vi "CRYPlot Data.vi"(6 "Down/Right Click?":bool=TRUE, 8 "Visible?":bool=TRUE, 9 "Rows":i32[](array[numeric]), 10 "Graph Type":string="XY", 11 "CurLib Tab Type":enum16{"Curves", "Values", "Results", "WFM"}(ring)) -> ()   [LabVIEW 2013]
uses:
  CRYWindow/DataView/SubVI/CRYData View Global.vi
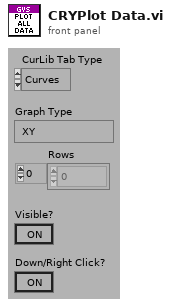
[diagram p1: front panel]
types:
  T1 = enum16{"OK", "Yes", "YesNo", "YesNoCancel", "ReplaceAppend"}
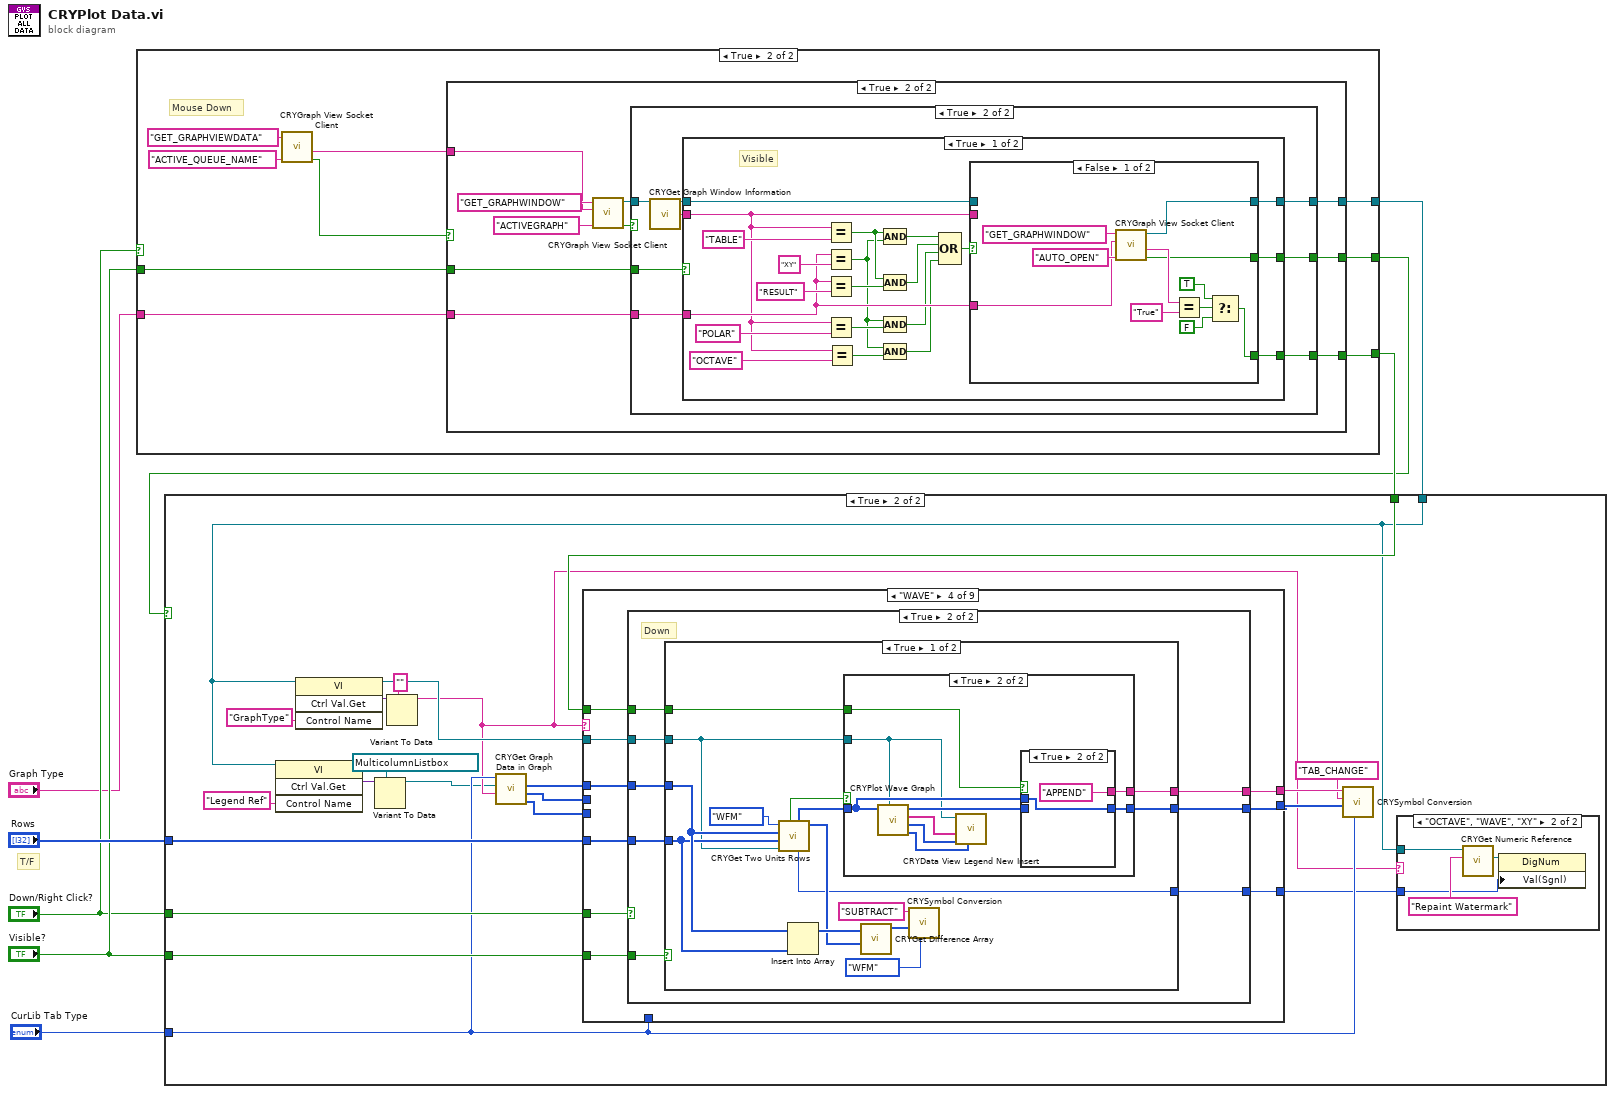
[diagram p0: block diagram]
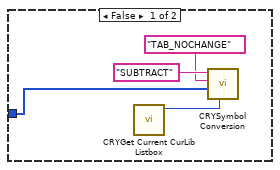
[diagram p2: hidden frame]
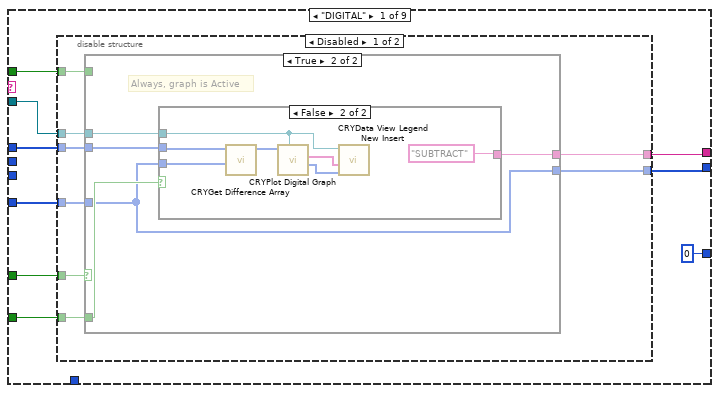
[diagram p4: hidden frame]
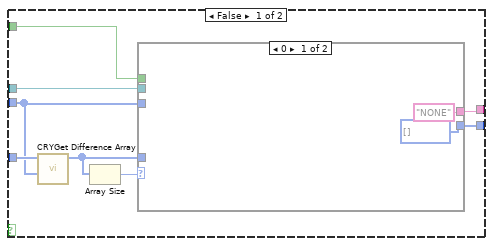
[diagram p5: hidden frame]
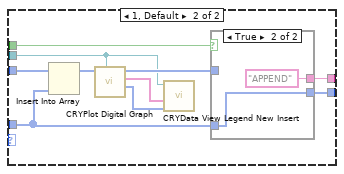
[diagram p6: hidden frame]
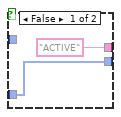
[diagram p7: hidden frame]
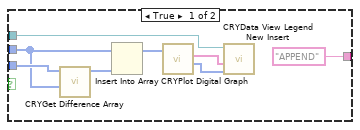
[diagram p8: hidden frame]
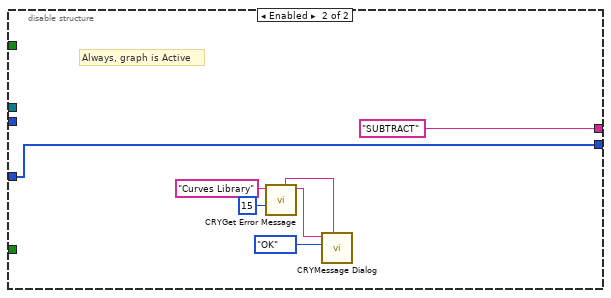
[diagram p9: hidden frame]
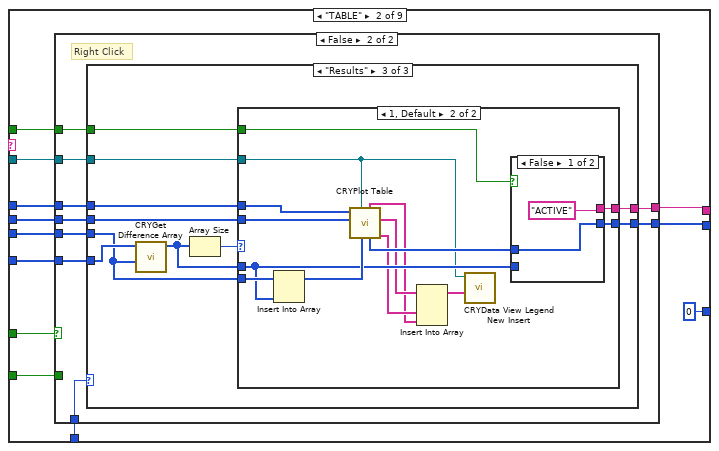
[diagram p10: hidden frame]
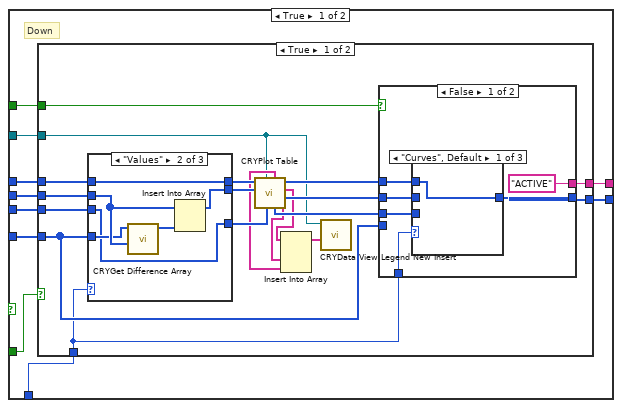
[diagram p11: hidden frame]
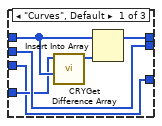
[diagram p12: hidden frame]
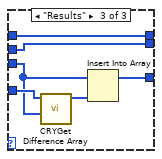
[diagram p13: hidden frame]
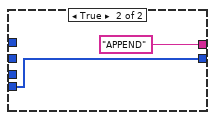
[diagram p16: hidden frame]
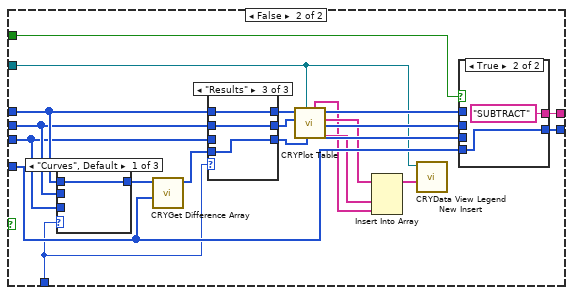
[diagram p17: hidden frame]
diagram:
  # "T/F"
  n1 = case shown="True" "Down/Right Click?" {
    tunnel: "Graph Type" -> [w9 w26]
    tunnel: [w11 w28] -> w5
    tunnel: "Visible?" -> [_ w29]
    tunnel: [w12 w27] -> w6
    tunnel: [w10 w22] -> w2
    frame False {
      # "Right Click"
      n2 = global write "CRYData View Global.vi" "Plot in Right Click?"(TRUE ("Plot in Right Click?")) -> ()
      n3 = call "CRYGraph View Socket Client.vi"("sOption"="AUTO_OPEN", "sData"=w9, "sAction"="GET_GRAPHWINDOW") -> ("bResult Out"=w10:bool, "sData Out"=w13:string, "pVI Out"=w11:refnum<vi>)  [unwired: 5 in, 1 out]
      n4 = Equal?(x=w13, y="True" ("sData Out")) -> (x = y?=w15:bool)
      n5 = Select(t=TRUE, s=w15, f=FALSE) -> (s? t:f=w12:bool)
    }
    frame True {
      # "Mouse Down"
      n6 = call "CRYGraph View Socket Client.vi"("sOption"="ACTIVE_QUEUE_NAME" ("sAction"), "sAction"="GET_GRAPHVIEWDATA") -> ("bResult Out"=w21:bool, "sData Out"=w23:string)  [unwired: 6 in, 2 out]
      n7 = case shown="True" w21 {
        tunnel: w29 -> [_ w50]
        tunnel: [w33 w46] -> w28
        tunnel: [w31 w45] -> w27
        tunnel: w26 -> [w30 w44]
        tunnel: w23 -> [_ w43]
        tunnel: [w32 w41] -> w22
        frame False {
          n8 = call "CRYGraph View Socket Client.vi"("sOption"="AUTO_OPEN", "sData"=w30, "sAction"="GET_GRAPHWINDOW") -> ("bResult Out"=w32:bool, "sData Out"=w34:string, "pVI Out"=w33:refnum<vi>)  [unwired: 5 in, 1 out]
          n9 = Equal?(x=w34, y="True" ("sData Out")) -> (x = y?=w37:bool)
          n10 = Select(t=TRUE, s=w37, f=FALSE) -> (s? t:f=w31:bool)
        }
        frame True {
          n11 = call "CRYGraph View Socket Client.vi"("sOption"="ACTIVEGRAPH", "sData"=w43, "sAction"="GET_GRAPHWINDOW") -> ("bResult Out"=w42:bool, "pVI Out"=w49:refnum<vi>)  [unwired: 5 in, 2 out]
          n12 = case shown="True" w42 {
            tunnel: w50 -> [_ w69]
            tunnel: w49 -> [_ w63]
            tunnel: w44 -> [w51 w67]
            tunnel: [w53 w66] -> w46
            tunnel: [w54 w64] -> w45
            tunnel: [w52 w62] -> w41
            frame False {
              n13 = call "CRYGraph View Socket Client.vi"("sOption"="AUTO_OPEN", "sData"=w51, "sAction"="GET_GRAPHWINDOW") -> ("bResult Out"=w52:bool, "sData Out"=w55:string, "pVI Out"=w53:refnum<vi>)  [unwired: 5 in, 1 out]
              n14 = Equal?(x=w55, y="True" ("sData Out")) -> (x = y?=w58:bool)
              n15 = Select(t=TRUE, s=w58, f=FALSE) -> (s? t:f=w54:bool)
            }
            frame True {
              n16 = call "CRYGet Graph Window Information.vi"("pGraph VI In"=w63) -> ("pGraph VI Out"=w68:refnum<vi>, "Graph Type Out"=w65:string)  [unwired: 2 in, 11 out]
              n17 = case shown="True" w69 {
                tunnel: w67 -> [w77 _]
                tunnel: w65 -> [w74 w107]
                tunnel: [w82 w112] -> w66
                tunnel: w68 -> [w83 w112]
                tunnel: [w81 TRUE] -> w64
                tunnel: [w80 TRUE ("bResult Out")] -> w62
                frame True {
                  # "Visible"
                  n18 = Equal?(x=w74, y="TABLE") -> (x = y?=w86:bool)
                  n19 = Equal?(x=w77, y="XY") -> (x = y?=w73:bool)
                  n20 = Equal?(x=w77, y="RESULT") -> (x = y?=w84:bool)
                  n21 = Equal?(x=w74, y="POLAR") -> (x = y?=w75:bool)
                  n22 = Equal?(x=w74, y="OCTAVE") -> (x = y?=w72:bool)
                  n23 = Compound Arithmetic op=AND(w86, w73) -> (w88:bool)
                  n24 = Compound Arithmetic op=AND(w86, w84) -> (w89:bool)
                  n25 = Compound Arithmetic op=AND(w73, w75) -> (w71:bool)
                  n26 = Compound Arithmetic op=AND(w73, w72) -> (w70:bool)
                  n27 = Compound Arithmetic op=OR(w88, w89, w71, w70) -> (w87:bool)
                  n28 = case shown="False" w87 {
                    tunnel: w77 -> [w91 _]
                    tunnel: [w93 w104] -> w82
                    tunnel: w83 -> [_ w104]
                    tunnel: [w94 w103] -> w81
                    tunnel: [w92 w103] -> w80
                    tunnel: w74 -> [_ w102]
                    frame False {
                      n29 = call "CRYGraph View Socket Client.vi"("sOption"="AUTO_OPEN", "sData"=w91, "sAction"="GET_GRAPHWINDOW") -> ("bResult Out"=w92:bool, "sData Out"=w98:string, "pVI Out"=w93:refnum<vi>)  [unwired: 5 in, 1 out]
                      n30 = Equal?(x=w98, y="True" ("sData Out")) -> (x = y?=w97:bool)
                      n31 = Select(t=TRUE, s=w97, f=FALSE) -> (s? t:f=w94:bool)
                    }
                    frame True {
                      w103 = TRUE
                      n32 = call "CRYGraph View Socket Client.vi"("sOption"="AUTO_OPEN", "sData"=w102, "sAction"="GET_GRAPHWINDOW") -> ()  [unwired: 5 in, 4 out]
                    }
                  }
                }
                frame False {
                  # "Surely, active Window is target to plot"
                  # "Invisible"
                  n33 = call "CRYGraph View Socket Client.vi"("sOption"="AUTO_OPEN", "sData"=w107, "sAction"="GET_GRAPHWINDOW") -> ()  [unwired: 5 in, 4 out]
                }
              }
            }
          }
        }
      }
    }
  }
  n34 = case shown="True" w2 {
    tunnel: "Rows" -> [w114 w138]
    tunnel: "Visible?" -> [_ w137]
    tunnel: w6 -> [_ w136]
    tunnel: w5 -> [_ w118]
    tunnel: "CurLib Tab Type" -> [_ w134]
    tunnel: "Down/Right Click?" -> [_ w135]
    frame False {
      n35 = call "CRYGet Current CurLib Listbox.vi"() -> ("Type"=w113:enum16{"Curves", "Values", "Results", "WFM"})  [unwired: 9 in, 2 out]
      n36 = call "CRYSymbol Conversion.vi"("CurLib Tab Type"=w113, "nDatas"=w114, "sData"="TAB_NOCHANGE" ("sActin"), "sActin"="SUBTRACT") -> ()  [unwired: 8 in]
    }
    frame True {
      n37 = invoke class="VI" method="Ctrl Val.Get"(reference=w118, "Control Name"="Legend Ref") -> ("Get Control Value Variant"=w120:variant)  [unwired: 2 in, 3 out]
      n38 = invoke class="VI" method="Ctrl Val.Get"(reference=w118, "Control Name"="GraphType") -> (reference out=w123:refnum<vi>, "Get Control Value Variant"=w124:variant)  [unwired: 2 in, 2 out]
      n39 = Variant To Data(type=refnum<vi> refnum ("GMListbox"), Variant=w120) -> (data=w117:refnum<vi>)  [unwired: 1 in, 1 out]
      n40 = Variant To Data(type="", Variant=w124) -> (data=w122:string)  [unwired: 1 in, 1 out]
      n41 = call "CRYGet Graph Data in Graph.vi"("Graph Type"=w122, "Legend Refnum"=w117, "Type In"=w134) -> ("Result Rows"=w131:i32[], "Value Rows"=w132:i32[], "Rows"=w133:i32[])  [unwired: 1 in, 5 out]
      n42 = case shown="\"WAVE\"" w122 {
        tunnel: w138 -> [w151 w222 w423 w487 w571 w636 w731 w830 _]
        tunnel: w133 -> [w150 w218 w424 w488 w572 w635 w730 w829 _]
        tunnel: w134 -> [_ w214 _ _ _ _ _ _ _]
        tunnel: w137 -> [w148 w219 w425 w489 w573 w632 w727 w826 _]
        tunnel: w135 -> [w149 w221 w422 w486 w570 w633 w728 w827 _]
        tunnel: w136 -> [w147 w220 w421 w485 _ w634 w729 w828 _]
        tunnel: [0 ("Two Units") 0 ("Two Units") 0 ("Two Units") w481 _ w631 w726 w825 0 ("Two Units")] -> w130
        tunnel: w132 -> [_ w217 _ _ _ _ _ _ _]
        tunnel: w131 -> [_ w215 _ _ _ _ _ _ _]
        tunnel: [w145 w213 w419 w484 w569 w630 w725 w824 "NONE" ("sActin")] -> w129
        tunnel: [w144 w212 w418 w483 w568 w629 w724 w823 i32[] [] ("Rows")] -> w128
        tunnel: w123 -> [w143 w211 w417 w482 w567 w628 w723 w822 _]
        frame "DIGITAL" {
          n43 = disable-structure shown="Disabled" {
            disable-tunnel: w151 -> [w159 w209]
            disable-tunnel: w150 -> [w158 _]
            disable-tunnel: w149 -> [w157 _]
            disable-tunnel: w148 -> [w156 _]
            disable-tunnel: w147 -> [w155 _]
            disable-tunnel: [w154 "SUBTRACT" ("sActin")] -> w145
            disable-tunnel: [w153 w209] -> w144
            disable-tunnel: w143 -> [w152 _]
            frame Disabled {
              n44 = case shown="True" w157 {
                tunnel: w159 -> [w165 w185]
                tunnel: w158 -> [w164 w188]
                tunnel: w156 -> [_ w187]
                tunnel: w155 -> [w163 _]
                tunnel: [w162 w186] -> w154
                tunnel: [w161 w185] -> w153
                tunnel: w152 -> [w160 w184]
                frame False {
                  n45 = call "CRYGet Difference Array.vi"("Array 2"=w164, "Array 1"=w165) -> ("Diff Out"=w167:i32[])  [unwired: 3 in, 6 out]
                  n46 = Array Size(array=w167) -> (size(s)=w166:i32)
                  n47 = case shown="0" w166 {
                    tunnel: w167 -> [_ w177]
                    tunnel: w164 -> [_ w179]
                    tunnel: w163 -> [_ w178]
                    tunnel: ["NONE" ("sActin") w172] -> w162
                    tunnel: [i32[] [] ("Rows") w171] -> w161
                    tunnel: w160 -> [_ w170]
                    frame 0 {
                    }
                    frame 1, Default {
                      n48 = Insert Into Array(array=w179, new element=w177) -> (w174:i32[])  [unwired: 1 in]
                      n49 = call "CRYPlot Digital Graph.vi"("pGraph VI In"=w170, "Selected Row In"=w174) -> ("Color Info"=w175:u32[], "Curve Name"=w176:string[], "Selected Row Out"=w173:i32[])  [unwired: 7 in]
                      n50 = call "CRYData View Legend New Insert.vi"("Color Array"=w175, "ItemName Array"=w176, "pGraph VI In"=w170) -> ()  [unwired: 2 in, 7 out]
                      n51 = case shown="True" w178 {
                        tunnel: w173 -> [_ _]
                        tunnel: w177 -> [w180 w182]
                        tunnel: ["ACTIVE" ("sActin") "APPEND" ("sActin")] -> w172
                        tunnel: [w180 w182] -> w171
                        frame False {
                        }
                        frame True {
                        }
                      }
                    }
                  }
                }
                frame True {
                  # "Always, graph is Active"
                  n52 = case shown="False" w187 {
                    tunnel: w185 -> [w195 w202]
                    tunnel: w188 -> [w194 w203]
                    tunnel: ["APPEND" ("sActin") "SUBTRACT" ("sActin")] -> w186
                    tunnel: w184 -> [w189 w197]
                    frame True {
                      n53 = call "CRYGet Difference Array.vi"("Array 2"=w194, "Array 1"=w195) -> ("Diff Out"=w196:i32[])  [unwired: 3 in, 6 out]
                      n54 = Insert Into Array(array=w194, new element=w196) -> (w191:i32[])  [unwired: 1 in]
                      n55 = call "CRYPlot Digital Graph.vi"("Selected Row In"=w191) -> ("Color Info"=w193:u32[], "Curve Name"=w192:string[])  [unwired: 8 in, 1 out]
                      n56 = call "CRYData View Legend New Insert.vi"("Color Array"=w193, "ItemName Array"=w192, "pGraph VI In"=w189) -> ()  [unwired: 2 in, 7 out]
                    }
                    frame False {
                      n57 = call "CRYGet Difference Array.vi"("Array 2"=w202, "Array 1"=w203) -> ("Diff Out"=w200:i32[])  [unwired: 3 in, 6 out]
                      n58 = call "CRYPlot Digital Graph.vi"("pGraph VI In"=w197, "Selected Row In"=w200) -> ("Color Info"=w199:u32[], "Curve Name"=w201:string[])  [unwired: 7 in, 1 out]
                      n59 = call "CRYData View Legend New Insert.vi"("Color Array"=w199, "ItemName Array"=w201, "pGraph VI In"=w197) -> ()  [unwired: 2 in, 7 out]
                    }
                  }
                }
              }
            }
            frame Enabled {
              # "Always, graph is Active"
              n60 = call "CRYGet Error Message.vi"("Error No"=15, "Kind"="Curves Library") -> ("Message"=w207:string, "Window Title"=w208:string)  [unwired: 4 in, 4 out]
              n61 = call "CRYMessage Dialog.vi"("Window Title"=w208, "YesNoCancel"=T1."OK", "Message Content"=w207) -> ()  [unwired: 7 in, 2 out]
            }
          }
        }
        frame "TABLE" {
          n62 = case shown="False" w221 {
            tunnel: w219 -> [w226 _]
            tunnel: w218 -> [w232 w325]
            tunnel: w222 -> [w230 w326]
            tunnel: w214 -> [w228 w323]
            tunnel: w220 -> [w231 w324]
            tunnel: w217 -> [w229 w322]
            tunnel: w215 -> [w227 w321]
            tunnel: [w225 w320] -> w213
            tunnel: [w224 w319] -> w212
            tunnel: w211 -> [w223 w318]
            frame True {
              # "Down"
              n63 = case shown="True" w226 {
                tunnel: w232 -> [w251 w301]
                tunnel: w231 -> [w250 w300]
                tunnel: w230 -> [w241 w298]
                tunnel: w229 -> [w248 w297]
                tunnel: w228 -> [w240 w286]
                tunnel: w227 -> [w246 w295]
                tunnel: [w239 w287] -> w224
                tunnel: [w238 w288] -> w225
                tunnel: w223 -> [w233 w281]
                frame True {
                  n64 = case shown="\"Values\"" w240 {
                    tunnel: w241 -> [w254 w260 w268]
                    tunnel: [w256 w263 w265] -> w243
                    tunnel: w248 -> [w256 w261 w265]
                    tunnel: [w257 w262 w269] -> w244
                    tunnel: w251 -> [w255 w262 w269]
                    tunnel: w246 -> [w252 w258 w266]
                    tunnel: [w252 w258 w264] -> w242
                    frame "Curves", Default {
                      n65 = call "CRYGet Difference Array.vi"("Array 2"=w255, "Array 1"=w254) -> ("Diff Out"=w253:i32[])  [unwired: 3 in, 6 out]
                      n66 = Insert Into Array(array=w255, new element=w253) -> (w257:i32[])  [unwired: 1 in]
                    }
                    frame "Values" {
                      n67 = call "CRYGet Difference Array.vi"("Array 2"=w261, "Array 1"=w260) -> ("Diff Out"=w259:i32[])  [unwired: 3 in, 6 out]
                      n68 = Insert Into Array(array=w261, new element=w259) -> (w263:i32[])  [unwired: 1 in]
                    }
                    frame "Results" {
                      n69 = call "CRYGet Difference Array.vi"("Array 2"=w266, "Array 1"=w268) -> ("Diff Out"=w267:i32[])  [unwired: 3 in, 6 out]
                      n70 = Insert Into Array(array=w266, new element=w267) -> (w264:i32[])  [unwired: 1 in]
                    }
                  }
                  n71 = call "CRYPlot Table.vi"("Result Rows In"=w242, "pGraph VI In"=w233, "Value Rows In"=w243, "Curve Rows In"=w244) -> ("Value Name"=w235:string[], "Value Rows Out"=w247:i32[], "Curve Name"=w236:string[], "Curve Rows Out"=w249:i32[], "Result Rows Out"=w245:i32[], "Result Name"=w237:string[])  [unwired: 2 in]
                  n72 = Insert Into Array(array=w236, new element #1=w235, new element #2=w237) -> (w234:string[])  [unwired: 1 in]
                  n73 = call "CRYData View Legend New Insert.vi"("ItemName Array"=w234, "pGraph VI In"=w233) -> ()  [unwired: 3 in, 7 out]
                  n74 = case shown="False" w250 {
                    tunnel: w240 -> [w274 _]
                    tunnel: w241 -> [_ w279]
                    tunnel: w249 -> [w275 _]
                    tunnel: w247 -> [w272 _]
                    tunnel: w245 -> [w273 _]
                    tunnel: [w271 w279] -> w239
                    tunnel: ["ACTIVE" ("sActin") "APPEND" ("sActin")] -> w238
                    frame False {
                      n75 = case shown="\"Curves\", Default" w274 {
                        tunnel: w275 -> [w276 _ _]
                        tunnel: w273 -> [_ _ w278]
                        tunnel: w272 -> [_ w277 _]
                        tunnel: [w276 w277 w278] -> w271
                        frame "Curves", Default {
                        }
                        frame "Values" {
                        }
                        frame "Results" {
                        }
                      }
                    }
                    frame True {
                    }
                  }
                }
                frame False {
                  n76 = case shown="\"Curves\", Default" w286 {
                    tunnel: w301 -> [w311 _ _]
                    tunnel: w297 -> [_ w312 _]
                    tunnel: w295 -> [_ _ w313]
                    tunnel: [w311 w312 w313] -> w293
                    frame "Curves", Default {
                    }
                    frame "Values" {
                    }
                    frame "Results" {
                    }
                  }
                  n77 = call "CRYGet Difference Array.vi"("Array 2"=w298, "Array 1"=w293) -> ("Diff Out"=w292:i32[])  [unwired: 3 in, 6 out]
                  n78 = case shown="\"Results\"" w286 {
                    tunnel: w301 -> [_ w306 w309]
                    tunnel: w297 -> [w303 _ w308]
                    tunnel: w295 -> [w302 w305 _]
                    tunnel: [w304 w306 w309] -> w291
                    tunnel: w292 -> [w304 w307 w310]
                    tunnel: [w303 w307 w308] -> w290
                    tunnel: [w302 w305 w310] -> w289
                    frame "Curves", Default {
                    }
                    frame "Values" {
                    }
                    frame "Results" {
                    }
                  }
                  n79 = call "CRYPlot Table.vi"("Result Rows In"=w289, "pGraph VI In"=w281, "Value Rows In"=w290, "Curve Rows In"=w291) -> ("Value Name"=w284:string[], "Value Rows Out"=w296:i32[], "Curve Name"=w285:string[], "Curve Rows Out"=w299:i32[], "Result Rows Out"=w294:i32[], "Result Name"=w283:string[])  [unwired: 2 in]
                  n80 = Insert Into Array(array=w285, new element #1=w284, new element #2=w283) -> (w282:string[])  [unwired: 1 in]
                  n81 = call "CRYData View Legend New Insert.vi"("ItemName Array"=w282, "pGraph VI In"=w281) -> ()  [unwired: 3 in, 7 out]
                  n82 = case shown="True" w300 {
                    tunnel: w298 -> [_ w316]
                    tunnel: w299 -> [_ _]
                    tunnel: w296 -> [_ _]
                    tunnel: w294 -> [_ _]
                    tunnel: ["NONE" ("sActin") "SUBTRACT" ("sActin")] -> w288
                    tunnel: [i32[] [] ("Rows") w316] -> w287
                    frame False {
                    }
                    frame True {
                    }
                  }
                }
              }
            }
            frame False {
              # "Right Click"
              n83 = case shown="\"Results\"" w323 {
                tunnel: w326 -> [w334 w364 w391]
                tunnel: w325 -> [w333 w361 w394]
                tunnel: w324 -> [w332 w363 w395]
                tunnel: w322 -> [w331 w362 w393]
                tunnel: w321 -> [w330 w360 w390]
                tunnel: [w329 w359 w389] -> w320
                tunnel: [w328 w358 w388] -> w319
                tunnel: w318 -> [w327 w357 w387]
                frame "Curves", Default {
                  n84 = call "CRYGet Difference Array.vi"("Array 2"=w333, "Array 1"=w334) -> ("Diff Out"=w335:i32[])  [unwired: 3 in, 6 out]
                  n85 = Array Size(array=w335) -> (size(s)=w336:i32)
                  n86 = case shown="1, Default" w336 {
                    tunnel: w333 -> [_ w349]
                    tunnel: w335 -> [_ w350]
                    tunnel: w332 -> [_ w351]
                    tunnel: w331 -> [_ w347]
                    tunnel: w330 -> [_ w346]
                    tunnel: ["NONE" ("sActin") w345] -> w329
                    tunnel: [i32[] [] ("Rows") w344] -> w328
                    tunnel: w327 -> [_ w339]
                    frame 0 {
                    }
                    frame 1, Default {
                      n87 = Insert Into Array(array=w349, new element=w350) -> (w348:i32[])  [unwired: 1 in]
                      n88 = call "CRYPlot Table.vi"("Result Rows In"=w346, "pGraph VI In"=w339, "Value Rows In"=w347, "Curve Rows In"=w348) -> ("Value Name"=w341:string[], "Curve Name"=w342:string[], "Curve Rows Out"=w352:i32[], "Result Name"=w340:string[])  [unwired: 2 in, 2 out]
                      n89 = Insert Into Array(array=w342, new element #1=w341, new element #2=w340) -> (w343:string[])  [unwired: 1 in]
                      n90 = call "CRYData View Legend New Insert.vi"("ItemName Array"=w343, "pGraph VI In"=w339) -> ()  [unwired: 3 in, 7 out]
                      n91 = case shown="False" w351 {
                        tunnel: w352 -> [w353 _]
                        tunnel: w350 -> [_ w355]
                        tunnel: ["ACTIVE" ("sActin") "APPEND" ("sActin")] -> w345
                        tunnel: [w353 w355] -> w344
                        frame False {
                        }
                        frame True {
                        }
                      }
                    }
                  }
                }
                frame "Values" {
                  n92 = call "CRYGet Difference Array.vi"("Array 2"=w362, "Array 1"=w364) -> ("Diff Out"=w365:i32[])  [unwired: 3 in, 6 out]
                  n93 = Array Size(array=w365) -> (size(s)=w366:i32)
                  n94 = case shown="1, Default" w366 {
                    tunnel: w362 -> [_ w380]
                    tunnel: w365 -> [_ w381]
                    tunnel: w363 -> [_ w382]
                    tunnel: w361 -> [_ w378]
                    tunnel: w360 -> [_ w376]
                    tunnel: ["NONE" ("sActin") w375] -> w359
                    tunnel: [i32[] [] ("Rows") w374] -> w358
                    tunnel: w357 -> [_ w369]
                    frame 0 {
                    }
                    frame 1, Default {
                      n95 = Insert Into Array(array=w380, new element=w381) -> (w379:i32[])  [unwired: 1 in]
                      n96 = call "CRYPlot Table.vi"("Result Rows In"=w376, "pGraph VI In"=w369, "Value Rows In"=w379, "Curve Rows In"=w378) -> ("Value Name"=w371:string[], "Value Rows Out"=w377:i32[], "Curve Name"=w372:string[], "Result Name"=w370:string[])  [unwired: 2 in, 2 out]
                      n97 = Insert Into Array(array=w372, new element #1=w371, new element #2=w370) -> (w373:string[])  [unwired: 1 in]
                      n98 = call "CRYData View Legend New Insert.vi"("ItemName Array"=w373, "pGraph VI In"=w369) -> ()  [unwired: 3 in, 7 out]
                      n99 = case shown="False" w382 {
                        tunnel: w381 -> [_ w385]
                        tunnel: w377 -> [w383 _]
                        tunnel: ["ACTIVE" ("sActin") "APPEND" ("sActin")] -> w375
                        tunnel: [w383 w385] -> w374
                        frame False {
                        }
                        frame True {
                        }
                      }
                    }
                  }
                }
                frame "Results" {
                  n100 = call "CRYGet Difference Array.vi"("Array 2"=w390, "Array 1"=w391) -> ("Diff Out"=w392:i32[])  [unwired: 3 in, 6 out]
                  n101 = Array Size(array=w392) -> (size(s)=w396:i32)
                  n102 = case shown="1, Default" w396 {
                    tunnel: w392 -> [_ w406]
                    tunnel: w395 -> [_ w412]
                    tunnel: w394 -> [_ w411]
                    tunnel: w393 -> [_ w410]
                    tunnel: w390 -> [_ w409]
                    tunnel: ["NONE" ("sActin") w405] -> w389
                    tunnel: [i32[] [] ("Rows") w404] -> w388
                    tunnel: w387 -> [_ w399]
                    frame 0 {
                    }
                    frame 1, Default {
                      n103 = Insert Into Array(array=w409, new element=w406) -> (w408:i32[])  [unwired: 1 in]
                      n104 = call "CRYPlot Table.vi"("Result Rows In"=w408, "pGraph VI In"=w399, "Value Rows In"=w410, "Curve Rows In"=w411) -> ("Value Name"=w401:string[], "Curve Name"=w402:string[], "Result Rows Out"=w407:i32[], "Result Name"=w400:string[])  [unwired: 2 in, 2 out]
                      n105 = Insert Into Array(array=w402, new element #1=w401, new element #2=w400) -> (w403:string[])  [unwired: 1 in]
                      n106 = call "CRYData View Legend New Insert.vi"("ItemName Array"=w403, "pGraph VI In"=w399) -> ()  [unwired: 3 in, 7 out]
                      n107 = case shown="False" w412 {
                        tunnel: w407 -> [w413 _]
                        tunnel: w406 -> [_ w415]
                        tunnel: ["ACTIVE" ("sActin") "APPEND" ("sActin")] -> w405
                        tunnel: [w413 w415] -> w404
                        frame False {
                        }
                        frame True {
                        }
                      }
                    }
                  }
                }
              }
            }
          }
        }
        frame "RESULT" {
          n108 = case shown="True" w422 {
            tunnel: w425 -> [_ w449]
            tunnel: w424 -> [w431 w454]
            tunnel: w423 -> [w430 w452]
            tunnel: w421 -> [w429 w453]
            tunnel: [w427 w451] -> w418
            tunnel: [w428 w450] -> w419
            tunnel: w417 -> [w426 w448]
            frame False {
              n109 = call "CRYGet Difference Array.vi"("Array 2"=w431, "Array 1"=w430) -> ("Diff Out"=w433:i32[])  [unwired: 3 in, 6 out]
              n110 = Array Size(array=w433) -> (size(s)=w432:i32)
              n111 = case shown="1, Default" w432 {
                tunnel: w431 -> [_ w441]
                tunnel: w433 -> [_ w440]
                tunnel: w429 -> [_ w442]
                tunnel: ["NONE" ("sActin") w439] -> w428
                tunnel: [i32[] [] ("Rows") w438] -> w427
                tunnel: w426 -> [_ w436]
                frame 0 {
                }
                frame 1, Default {
                  n112 = call "CRYPlot Result.vi"("pGraph VI In"=w436, "New Rows In"=w440, "Old Rows In"=w441) -> ("Curve Name"=w437:string[], "Selected Rows Out"=w443:i32[])  [unwired: 2 in, 5 out]
                  n113 = call "CRYData View Legend New Insert.vi"("ItemName Array"=w437, "pGraph VI In"=w436) -> ()  [unwired: 3 in, 7 out]
                  n114 = case shown="False" w442 {
                    tunnel: w443 -> [w444 _]
                    tunnel: w440 -> [_ w446]
                    tunnel: ["ACTIVE" ("sActin") "APPEND" ("sActin")] -> w439
                    tunnel: [w444 w446] -> w438
                    frame False {
                    }
                    frame True {
                    }
                  }
                }
              }
            }
            frame True {
              # "Down"
              n115 = case shown="False" w449 {
                tunnel: w454 -> [w462 w475]
                tunnel: w453 -> [w461 w474]
                tunnel: w452 -> [w460 w473]
                tunnel: [w459 w472] -> w451
                tunnel: [w458 w471] -> w450
                tunnel: w448 -> [w455 w469]
                frame True {
                  n116 = call "CRYGet Difference Array.vi"("Array 2"=w462, "Array 1"=w460) -> ("Diff Out"=w457:i32[])  [unwired: 3 in, 6 out]
                  n117 = Insert Into Array(array=w462, new element=w457) -> (w464:i32[])  [unwired: 1 in]
                  n118 = call "CRYPlot Result.vi"("pGraph VI In"=w455, "Old Rows In"=w464) -> ("Curve Name"=w456:string[], "Selected Rows Out"=w463:i32[])  [unwired: 3 in, 5 out]
                  n119 = call "CRYData View Legend New Insert.vi"("ItemName Array"=w456, "pGraph VI In"=w455) -> ()  [unwired: 3 in, 7 out]
                  n120 = case shown="True" w461 {
                    tunnel: w463 -> [w466 _]
                    tunnel: [w466 w467] -> w459
                    tunnel: ["ACTIVE" ("sActin") "APPEND" ("sActin")] -> w458
                    tunnel: w460 -> [_ w467]
                    frame False {
                    }
                    frame True {
                    }
                  }
                }
                frame False {
                  # "Invisible"
                  n121 = call "CRYGet Difference Array.vi"("Array 2"=w473, "Array 1"=w475) -> ("Diff Out"=w476:i32[])  [unwired: 3 in, 6 out]
                  n122 = call "CRYPlot Result.vi"("pGraph VI In"=w469, "Old Rows In"=w476) -> ("Curve Name"=w470:string[])  [unwired: 3 in, 6 out]
                  n123 = call "CRYData View Legend New Insert.vi"("ItemName Array"=w470, "pGraph VI In"=w469) -> ()  [unwired: 3 in, 7 out]
                  n124 = case shown="True" w474 {
                    tunnel: [i32[] [] ("Rows") w479] -> w472
                    tunnel: ["NONE" ("sActin") "SUBTRACT" ("sActin")] -> w471
                    tunnel: w473 -> [_ w479]
                    frame False {
                    }
                    frame True {
                    }
                  }
                }
              }
            }
          }
        }
        frame "WAVE" {
          n125 = case shown="True" w486 {
            tunnel: w489 -> [_ w517]
            tunnel: w488 -> [w493 w522]
            tunnel: w487 -> [w492 w520]
            tunnel: w485 -> [w499 w521]
            tunnel: [w498 w519] -> w483
            tunnel: [w497 w518] -> w484
            tunnel: w482 -> [w490 w516]
            tunnel: [w491 w515] -> w481
            frame False {
              n126 = call "CRYGet Two Units Rows.vi"("pGraph VI In"=w490, "New Rows In"=w492, "Old Rows In"=w493, "Type"=enum16{"Curves", "Values", "Results", "WFM"}."WFM") -> ("Two Units"=w491:i32, "New Rows Out"=w495:i32[], "New Exist?"=w496:bool)  [unwired: 1 in, 4 out]
              n127 = case shown="True" w496 {
                tunnel: w493 -> [_ _]
                tunnel: w495 -> [w502 _]
                tunnel: w499 -> [w505 _]
                tunnel: [w503 i32[] [] ("Rows")] -> w498
                tunnel: [w504 "NONE" ("sActin")] -> w497
                tunnel: w490 -> [w500 _]
                frame True {
                  n128 = call "CRYPlot Wave Graph.vi"("pGraph VI In"=w500, "Selected Rows In"=w502) -> ("ItemSyms"=w501:i32[], "Color Info"=w508:u32[], "Curve Name"=w507:string[], "Selected Rows Out"=w506:i32[])  [unwired: 3 in, 3 out]
                  n129 = call "CRYData View Legend New Insert.vi"("Item Symbols"=w501, "Color Array"=w508, "ItemName Array"=w507, "pGraph VI In"=w500) -> ()  [unwired: 1 in, 7 out]
                  n130 = case shown="False" w505 {
                    tunnel: w506 -> [w509 _]
                    tunnel: w502 -> [_ w511]
                    tunnel: ["ACTIVE" ("sActin") "APPEND" ("sActin")] -> w504
                    tunnel: [w509 w511] -> w503
                    frame False {
                    }
                    frame True {
                    }
                  }
                }
                frame False {
                }
              }
            }
            frame True {
              # "Down"
              n131 = case shown="True" w517 {
                tunnel: w522 -> [w528 w556]
                tunnel: w521 -> [w537 _]
                tunnel: w520 -> [w527 w555]
                tunnel: [w536 i32[] [] ("Rows")] -> w519
                tunnel: [w535 "NONE" ("sActin")] -> w518
                tunnel: w516 -> [w524 w559]
                tunnel: [w525 0 ("Two Units")] -> w515
                frame True {
                  n132 = call "CRYGet Two Units Rows.vi"("pGraph VI In"=w524, "New Rows In"=w527, "Old Rows In"=w528, "Type"=enum16{"Curves", "Values", "Results", "WFM"}."WFM") -> ("All Rows Out"=w526:i32[], "Two Units"=w525:i32, "New Rows Out"=w533:i32[], "New Exist?"=w534:bool)  [unwired: 1 in, 3 out]
                  n133 = Insert Into Array(array=w528, new element=w527) -> (w529:i32[])  [unwired: 1 in]
                  n134 = case shown="True" w534 {
                    tunnel: w537 -> [_ w545]
                    tunnel: [i32[] [] ("New Rows Out") w544] -> w536
                    tunnel: ["NONE" ("sActin") w543] -> w535
                    tunnel: w533 -> [_ w541]
                    tunnel: w524 -> [_ w540]
                    frame False {
                    }
                    frame True {
                      n135 = call "CRYPlot Wave Graph.vi"("pGraph VI In"=w540, "Selected Rows In"=w541) -> ("ItemSyms"=w542:i32[], "Color Info"=w546:u32[], "Curve Name"=w547:string[], "Selected Rows Out"=w548:i32[])  [unwired: 3 in, 3 out]
                      n136 = call "CRYData View Legend New Insert.vi"("Item Symbols"=w542, "Color Array"=w546, "ItemName Array"=w547, "pGraph VI In"=w540) -> ()  [unwired: 1 in, 7 out]
                      n137 = case shown="True" w545 {
                        tunnel: w548 -> [w550 _]
                        tunnel: [w550 w551] -> w544
                        tunnel: ["ACTIVE" ("sActin") "APPEND" ("sActin")] -> w543
                        tunnel: w541 -> [_ w551]
                        frame False {
                        }
                        frame True {
                        }
                      }
                    }
                  }
                  n138 = call "CRYGet Difference Array.vi"("Array 2"=w526, "Array 1"=w529) -> ("Diff Out"=w530:i32[])  [unwired: 3 in, 6 out]
                  n139 = call "CRYSymbol Conversion.vi"("CurLib Tab Type"=enum16{"Curves", "Values", "Results", "WFM"}."WFM", "nDatas"=w530, "sActin"="SUBTRACT") -> ()  [unwired: 9 in]
                }
                frame False {
                  # "Invisible"
                  n140 = Index Array(array=w555) -> (element=w562:i32)  [unwired: 1 in]
                  n141 = Search 1D Array(1D array=w556, element=w562) -> (index of element=w560:i32)  [unwired: 1 in]
                  n142 = Build Array(w560) -> (w553:i32[])
                  n143 = invoke class="VI" method="Ctrl Val.Set"(reference=w559, "Control Name"="SelectedRow", "Value"=w553) -> (reference out=w566:refnum<vi>)  [unwired: 2 in, 4 out]
                  n144 = call "CRYGet Boolean Reference.vi"("Label Name"="RemoveSome", "VI Refnum"=w566) -> ("Boolean Ref"=w564:refnum<vi>)  [unwired: 7 in, 2 out]
                  n145 = property class="Bool"(reference=w564, "Val(Sgnl)"=TRUE) -> ()  [unwired: 1 in, 2 out]
                }
              }
            }
          }
        }
        frame "INTENSITY" {
          n146 = case shown="True" w570 {
            tunnel: w573 -> [_ w593]
            tunnel: w572 -> [w577 w597]
            tunnel: w571 -> [w578 w596]
            tunnel: [w580 w595] -> w568
            tunnel: [w579 w594] -> w569
            tunnel: w567 -> [w574 w592]
            frame False {
              n147 = call "CRYGet Difference Array.vi"("Array 2"=w577, "Array 1"=w578) -> ("Diff Out"=w575:i32[])  [unwired: 3 in, 6 out]
              n148 = Array Size(array=w575) -> (size(s)=w576:i32)
              n149 = case shown="1, Default" w576 {
                tunnel: [i32[] [] ("All Rows Out") w591] -> w580
                tunnel: ["NONE" ("sActin") "ACTIVE" ("sActin")] -> w579
                tunnel: w577 -> [_ w585]
                tunnel: w575 -> [_ w584]
                tunnel: w574 -> [_ w583]
                frame 0 {
                }
                frame 1, Default {
                  n150 = Insert Into Array(array=w585, new element=w584) -> (w586:i32[])  [unwired: 1 in]
                  n151 = call "CRYPlot Intensity Graph.vi"("pGraph VI In"=w583, "Selected Rows In"=w586) -> ("ItemSyms"=w587:i32[], "Color Info"=w589:u32[], "Wave Names"=w588:string[], "All Rows Out"=w591:i32[])  [unwired: 6 in]
                  n152 = call "CRYData View Legend New Insert.vi"("Item Symbols"=w587, "Color Array"=w589, "ItemName Array"=w588, "pGraph VI In"=w583) -> ()  [unwired: 1 in, 7 out]
                }
              }
            }
            frame True {
              # "Down"
              n153 = case shown="True" w593 {
                tunnel: w597 -> [w601 w618]
                tunnel: w596 -> [w602 w617]
                tunnel: [w604 i32[] [] ("Rows")] -> w595
                tunnel: [w603 "NONE" ("sActin")] -> w594
                tunnel: w592 -> [w598 w621]
                frame True {
                  n154 = call "CRYGet Difference Array.vi"("Array 2"=w601, "Array 1"=w602) -> ("Diff Out"=w599:i32[])  [unwired: 3 in, 6 out]
                  n155 = Array Size(array=w599) -> (size(s)=w600:i32)
                  n156 = case shown="1, Default" w600 {
                    tunnel: [i32[] [] ("All Rows Out") w615] -> w604
                    tunnel: ["NONE" ("sActin") "ACTIVE" ("sActin")] -> w603
                    tunnel: w601 -> [_ w613]
                    tunnel: w599 -> [_ w612]
                    tunnel: w598 -> [_ w607]
                    frame 0 {
                    }
                    frame 1, Default {
                      n157 = Insert Into Array(array=w613, new element=w612) -> (w611:i32[])  [unwired: 1 in]
                      n158 = call "CRYPlot Intensity Graph.vi"("pGraph VI In"=w607, "Selected Rows In"=w611) -> ("ItemSyms"=w608:i32[], "Color Info"=w609:u32[], "Wave Names"=w610:string[], "All Rows Out"=w615:i32[])  [unwired: 6 in]
                      n159 = call "CRYData View Legend New Insert.vi"("Item Symbols"=w608, "Color Array"=w609, "ItemName Array"=w610, "pGraph VI In"=w607) -> ()  [unwired: 1 in, 7 out]
                    }
                  }
                }
                frame False {
                  # "Invisible"
                  n160 = Index Array(array=w617) -> (element=w623:i32)  [unwired: 1 in]
                  n161 = Search 1D Array(1D array=w618, element=w623) -> (index of element=w616:i32)  [unwired: 1 in]
                  n162 = invoke class="VI" method="Ctrl Val.Set"(reference=w621, "Control Name"="OldRow", "Value"=w616) -> (reference out=w627:refnum<vi>)  [unwired: 2 in, 4 out]
                  n163 = call "CRYGet Boolean Reference.vi"("Label Name"="RemoveOne", "VI Refnum"=w627) -> ("Boolean Ref"=w625:refnum<vi>)  [unwired: 7 in, 2 out]
                  n164 = property class="Bool"(reference=w625, "Val(Sgnl)"=TRUE) -> ()  [unwired: 1 in, 2 out]
                }
              }
            }
          }
        }
        frame "XY" {
          n165 = case shown="True" w633 {
            tunnel: w636 -> [w642 w703]
            tunnel: w635 -> [w643 w702]
            tunnel: w634 -> [w641 w707]
            tunnel: w632 -> [w644 _]
            tunnel: [w640 w701] -> w631
            tunnel: [w639 w700] -> w630
            tunnel: [w638 w699] -> w629
            tunnel: w628 -> [w637 w698]
            frame True {
              # "Down"
              n166 = case shown="True" w644 {
                tunnel: w643 -> [w648 w684]
                tunnel: w642 -> [w647 w690]
                tunnel: w641 -> [w657 _]
                tunnel: [w654 w697] -> w640
                tunnel: [w653 "NONE" ("sActin")] -> w639
                tunnel: [w652 i32[] [] ("Rows")] -> w638
                tunnel: w637 -> [w645 w674]
                frame True {
                  n167 = call "CRYGet Two Units Rows.vi"("pGraph VI In"=w645, "New Rows In"=w647, "Old Rows In"=w648) -> ("All Rows Out"=w646:i32[], "Two Units"=w654:i32, "New Rows Out"=w655:i32[], "New Exist?"=w656:bool)  [unwired: 2 in, 3 out]
                  n168 = Insert Into Array(array=w648, new element=w647) -> (w649:i32[])  [unwired: 1 in]
                  n169 = call "CRYGet Difference Array.vi"("Array 2"=w646, "Array 1"=w649) -> ("Diff Out"=w650:i32[])  [unwired: 3 in, 6 out]
                  n170 = case shown="True" w656 {
                    tunnel: w657 -> [w664 _]
                    tunnel: w655 -> [w660 _]
                    tunnel: w647 -> [_ _]
                    tunnel: [w662 "NONE" ("sActin")] -> w653
                    tunnel: [w661 i32[] [] ("New Rows Out")] -> w652
                    tunnel: w645 -> [w658 _]
                    frame True {
                      n171 = call "CRYPlot XY Graph.vi"("pGraph VI In"=w658, "Selected Rows In"=w660) -> ("Color Info"=w666:u32[], "Curve Name"=w665:string[], "All Rows Out"=w663:i32[], "ItemSyms"=w659:i32[])  [unwired: 4 in, 2 out]
                      n172 = call "CRYData View Legend New Insert.vi"("Item Symbols"=w659, "Color Array"=w666, "ItemName Array"=w665, "pGraph VI In"=w658) -> ()  [unwired: 1 in, 7 out]
                      n173 = case shown="False" w664 {
                        tunnel: w663 -> [w668 _]
                        tunnel: w660 -> [_ w669]
                        tunnel: ["ACTIVE" ("sActin") "APPEND" ("sActin")] -> w662
                        tunnel: [w668 w669] -> w661
                        frame False {
                        }
                        frame True {
                        }
                      }
                    }
                    frame False {
                    }
                  }
                  n174 = call "CRYSymbol Conversion.vi"("nDatas"=w650, "sActin"="SUBTRACT") -> ()  [unwired: 10 in]
                }
                frame False {
                  n175 = Index Array(array=w690) -> (element=w689:i32)  [unwired: 1 in]
                  n176 = invoke class="VI" method="Ctrl Val.Get"(reference=w674, "Control Name"="MagnitudeShow") -> ("Get Control Value Variant"=w676:variant)  [unwired: 2 in, 3 out]
                  n177 = invoke class="VI" method="Ctrl Val.Get"(reference=w674, "Control Name"="PhaseShow") -> ("Get Control Value Variant"=w679:variant)  [unwired: 2 in, 3 out]
                  n178 = Variant To Data(type=TRUE, Variant=w676) -> (data=w681:bool)  [unwired: 1 in, 1 out]
                  n179 = Variant To Data(type=TRUE, Variant=w679) -> (data=w682:bool)  [unwired: 1 in, 1 out]
                  n180 = And(x=w681, y=w682) -> (x .and. y?=w673:bool)
                  n181 = call "CRYMake Phase Index.vi"("Mag_Phase Flag"=w673, "Selected Rows In"=w684) -> ("Selected Rows Out"=w683:i32[])  [unwired: 8 in, 1 out]
                  n182 = Search 1D Array(1D array=w683, element=w689) -> (index of element=w687:i32)  [unwired: 1 in]
                  n183 = Build Array(w687) -> (w685:i32[])
                  n184 = invoke class="VI" method="Ctrl Val.Set"(reference=w674, "Control Name"="SelectedRow", "Value"=w685) -> (reference out=w694:refnum<vi>)  [unwired: 2 in, 4 out]
                  n185 = Delete From Array(array=w683, index=w687) -> (array with subset deleted=w686:i32[])  [unwired: 1 in, 1 out]
                  n186 = call "CRYGet Two Units Rows.vi"("pGraph VI In"=w674, "Old Rows In"=w686) -> ("Two Units"=w697:i32)  [unwired: 3 in, 6 out]
                  n187 = call "CRYGet Boolean Reference.vi"("Label Name"="RemoveSome", "VI Refnum"=w694) -> ("Boolean Ref"=w692:refnum<vi>)  [unwired: 7 in, 2 out]
                  n188 = property class="Bool"(reference=w692, "Val(Sgnl)"=TRUE) -> ()  [unwired: 1 in, 2 out]
                }
              }
            }
            frame False {
              n189 = call "CRYGet Difference Array.vi"("Array 2"=w702, "Array 1"=w703) -> ("Diff Out"=w704:i32[])  [unwired: 3 in, 6 out]
              n190 = call "CRYGet Two Units Rows.vi"("pGraph VI In"=w698, "New Rows In"=w704, "Old Rows In"=w702) -> ("Two Units"=w701:i32, "New Rows Out"=w705:i32[], "New Exist?"=w706:bool)  [unwired: 2 in, 4 out]
              n191 = case shown="True" w706 {
                tunnel: w707 -> [_ w718]
                tunnel: w705 -> [_ w712]
                tunnel: ["NONE" ("sActin") w714] -> w700
                tunnel: [i32[] [] ("All Rows Out") w713] -> w699
                tunnel: w698 -> [_ w710]
                frame False {
                }
                frame True {
                  n192 = call "CRYPlot XY Graph.vi"("pGraph VI In"=w710, "Selected Rows In"=w712) -> ("Color Info"=w717:u32[], "Curve Name"=w716:string[], "All Rows Out"=w715:i32[], "ItemSyms"=w711:i32[])  [unwired: 4 in, 2 out]
                  n193 = call "CRYData View Legend New Insert.vi"("Item Symbols"=w711, "Color Array"=w717, "ItemName Array"=w716, "pGraph VI In"=w710) -> ()  [unwired: 1 in, 7 out]
                  n194 = case shown="False" w718 {
                    tunnel: w712 -> [w719 _]
                    tunnel: w715 -> [_ w722]
                    tunnel: ["APPEND" ("sActin") "ACTIVE" ("sActin")] -> w714
                    tunnel: [w719 w722] -> w713
                    frame True {
                    }
                    frame False {
                    }
                  }
                }
              }
            }
          }
        }
        frame "POLAR" {
          n195 = case shown="False" w728 {
            tunnel: w731 -> [w737 w797]
            tunnel: w730 -> [w738 w796]
            tunnel: w729 -> [w736 w801]
            tunnel: w727 -> [w739 _]
            tunnel: [w735 w795] -> w726
            tunnel: [w734 w794] -> w725
            tunnel: [w733 w793] -> w724
            tunnel: w723 -> [w732 w791]
            frame True {
              # "Down"
              n196 = case shown="False" w739 {
                tunnel: w738 -> [w743 w781]
                tunnel: w737 -> [w742 w784]
                tunnel: w736 -> [w752 _]
                tunnel: [w749 w790] -> w735
                tunnel: [w748 "NONE" ("sActin")] -> w734
                tunnel: [w747 i32[] [] ("Rows")] -> w733
                tunnel: w732 -> [w740 w775]
                frame True {
                  n197 = Insert Into Array(array=w743, new element=w742) -> (w744:i32[])  [unwired: 1 in]
                  n198 = call "CRYGet Two Units Rows.vi"("pGraph VI In"=w740, "New Rows In"=w742, "Old Rows In"=w743) -> ("All Rows Out"=w741:i32[], "Two Units"=w749:i32, "New Rows Out"=w750:i32[], "New Exist?"=w751:bool)  [unwired: 2 in, 3 out]
                  n199 = case shown="True" w751 {
                    tunnel: w752 -> [w764 _]
                    tunnel: w750 -> [w756 _]
                    tunnel: w742 -> [_ _]
                    tunnel: [w762 "NONE" ("sActin")] -> w748
                    tunnel: [w761 i32[] [] ("New Rows Out")] -> w747
                    tunnel: w741 -> [w755 _]
                    tunnel: w740 -> [w754 _]
                    frame True {
                      w753 = "POLAR_PlotXY" ("sOption")
                      n200 = call "CRYPlot XY Graph.vi"("pGraph VI In"=w754, "sType"=w753, "Selected Rows In"=w756) -> ("Color Info"=w766:u32[], "Curve Name"=w765:string[], "All Rows Out"=w763:i32[], "ItemSyms"=w760:i32[])  [unwired: 3 in, 2 out]
                      n201 = call "CRYData View Legend New Insert.vi"("Item Symbols"=w760, "Color Array"=w766, "ItemName Array"=w765, "sOption"=w753, "pGraph VI In"=w754) -> ()  [unwired: 7 out]
                      n202 = call "CRYPlot Polar Graph.vi"("pGraph VI In"=w754, "Selected Rows In"=w755) -> ("Freq Color"=w758:u32[], "Freq Name"=w757:string[])  [unwired: 4 in, 4 out]
                      n203 = case shown="True" w764 {
                        tunnel: w763 -> [w768 _]
                        tunnel: w756 -> [_ w769]
                        tunnel: ["ACTIVE" ("sActin") "APPEND" ("sActin")] -> w762
                        tunnel: [w768 w769] -> w761
                        frame False {
                        }
                        frame True {
                        }
                      }
                      n204 = call "CRYData View Legend New Insert.vi"("Color Array"=w758, "ItemName Array"=w757, "sOption"="POLAR_XY", "pGraph VI In"=w754) -> ()  [unwired: 1 in, 7 out]
                    }
                    frame False {
                    }
                  }
                  n205 = call "CRYGet Difference Array.vi"("Array 2"=w741, "Array 1"=w744) -> ("Diff Out"=w745:i32[])  [unwired: 3 in, 6 out]
                  n206 = call "CRYSymbol Conversion.vi"("nDatas"=w745, "sActin"="SUBTRACT") -> ()  [unwired: 10 in]
                }
                frame False {
                  n207 = Index Array(array=w784) -> (element=w783:i32)  [unwired: 1 in]
                  n208 = Search 1D Array(1D array=w781, element=w783) -> (index of element=w776:i32)  [unwired: 1 in]
                  n209 = Build Array(w776) -> (w774:i32[])
                  n210 = Delete From Array(array=w781, index=w776) -> (array with subset deleted=w777:i32[])  [unwired: 1 in, 1 out]
                  n211 = invoke class="VI" method="Ctrl Val.Set"(reference=w775, "Control Name"="SelectedRow", "Value"=w774) -> (reference out=w773:refnum<vi>)  [unwired: 2 in, 4 out]
                  n212 = call "CRYPlot Polar Graph.vi"("pGraph VI In"=w775, "Selected Rows In"=w777) -> ("Freq Color"=w779:u32[], "Freq Name"=w778:string[])  [unwired: 4 in, 4 out]
                  n213 = call "CRYGet Two Units Rows.vi"("pGraph VI In"=w773, "Old Rows In"=w777) -> ("Two Units"=w790:i32)  [unwired: 3 in, 6 out]
                  n214 = call "CRYData View Legend New Insert.vi"("Color Array"=w779, "ItemName Array"=w778, "sOption"="POLAR_XY", "pGraph VI In"=w775) -> ()  [unwired: 1 in, 7 out]
                  n215 = call "CRYGet Boolean Reference.vi"("Label Name"="RemoveSome", "VI Refnum"=w773) -> ("Boolean Ref"=w786:refnum<vi>)  [unwired: 7 in, 2 out]
                  n216 = property class="Bool"(reference=w786, "Val(Sgnl)"=TRUE) -> ()  [unwired: 1 in, 2 out]
                }
              }
            }
            frame False {
              n217 = call "CRYGet Difference Array.vi"("Array 2"=w796, "Array 1"=w797) -> ("Diff Out"=w798:i32[])  [unwired: 3 in, 6 out]
              n218 = call "CRYGet Two Units Rows.vi"("pGraph VI In"=w791, "New Rows In"=w798, "Old Rows In"=w796) -> ("All Rows Out"=w792:i32[], "Two Units"=w795:i32, "New Rows Out"=w799:i32[], "New Exist?"=w800:bool)  [unwired: 2 in, 3 out]
              n219 = case shown="True" w800 {
                tunnel: w801 -> [_ w817]
                tunnel: w799 -> [_ w811]
                tunnel: ["NONE" ("sActin") w813] -> w794
                tunnel: [i32[] [] ("All Rows Out") w812] -> w793
                tunnel: w792 -> [_ w806]
                tunnel: w791 -> [_ w805]
                frame False {
                }
                frame True {
                  w804 = "POLAR_PlotXY" ("sOption")
                  n220 = call "CRYPlot Polar Graph.vi"("pGraph VI In"=w805, "Selected Rows In"=w806) -> ("Freq Color"=w808:u32[], "Freq Name"=w807:string[])  [unwired: 4 in, 4 out]
                  n221 = call "CRYPlot XY Graph.vi"("pGraph VI In"=w805, "sType"=w804, "Selected Rows In"=w811) -> ("Color Info"=w816:u32[], "Curve Name"=w815:string[], "All Rows Out"=w814:i32[], "ItemSyms"=w810:i32[])  [unwired: 3 in, 2 out]
                  n222 = call "CRYData View Legend New Insert.vi"("Color Array"=w808, "ItemName Array"=w807, "sOption"="POLAR_XY", "pGraph VI In"=w805) -> ()  [unwired: 1 in, 7 out]
                  n223 = call "CRYData View Legend New Insert.vi"("Item Symbols"=w810, "Color Array"=w816, "ItemName Array"=w815, "sOption"=w804, "pGraph VI In"=w805) -> ()  [unwired: 7 out]
                  n224 = case shown="False" w817 {
                    tunnel: w811 -> [w818 _]
                    tunnel: w814 -> [_ w821]
                    tunnel: ["APPEND" ("sActin") "ACTIVE" ("sActin")] -> w813
                    tunnel: [w818 w821] -> w812
                    frame True {
                    }
                    frame False {
                    }
                  }
                }
              }
            }
          }
        }
        frame "OCTAVE" {
          n225 = case shown="True" w827 {
            tunnel: w830 -> [w836 w887]
            tunnel: w829 -> [w837 w886]
            tunnel: w828 -> [w835 w891]
            tunnel: w826 -> [w838 _]
            tunnel: [w834 w885] -> w825
            tunnel: [w833 w884] -> w824
            tunnel: [w832 w883] -> w823
            tunnel: w822 -> [w831 w882]
            frame True {
              # "Down"
              n226 = case shown="True" w838 {
                tunnel: w837 -> [w842 w870]
                tunnel: w836 -> [w841 w874]
                tunnel: w835 -> [w851 _]
                tunnel: [w848 w881] -> w834
                tunnel: [w847 "NONE" ("sActin")] -> w833
                tunnel: [w846 i32[] [] ("Rows")] -> w832
                tunnel: w831 -> [w839 w867]
                frame True {
                  n227 = call "CRYGet Two Units Rows.vi"("pGraph VI In"=w839, "New Rows In"=w841, "Old Rows In"=w842) -> ("All Rows Out"=w840:i32[], "Two Units"=w848:i32, "New Rows Out"=w849:i32[], "New Exist?"=w850:bool)  [unwired: 2 in, 3 out]
                  n228 = Insert Into Array(array=w842, new element=w841) -> (w843:i32[])  [unwired: 1 in]
                  n229 = case shown="True" w850 {
                    tunnel: w851 -> [w858 _]
                    tunnel: w849 -> [w854 _]
                    tunnel: w841 -> [_ _]
                    tunnel: [w856 "NONE" ("sActin")] -> w847
                    tunnel: [w855 i32[] [] ("New Rows Out")] -> w846
                    tunnel: w839 -> [w852 _]
                    frame True {
                      n230 = call "CRYPlot Octave Graph.vi"("pGraph VI In"=w852, "Selected Rows In"=w854) -> ("Color Info"=w860:u32[], "Curve Name"=w859:string[], "All Rows Out"=w857:i32[], "ItemSyms"=w853:i32[])  [unwired: 6 in]
                      n231 = call "CRYData View Legend New Insert.vi"("Item Symbols"=w853, "Color Array"=w860, "ItemName Array"=w859, "pGraph VI In"=w852) -> ()  [unwired: 1 in, 7 out]
                      n232 = case shown="False" w858 {
                        tunnel: w857 -> [w862 _]
                        tunnel: w854 -> [_ w863]
                        tunnel: ["ACTIVE" ("sActin") "APPEND" ("sActin")] -> w856
                        tunnel: [w862 w863] -> w855
                        frame False {
                        }
                        frame True {
                        }
                      }
                    }
                    frame False {
                    }
                  }
                  n233 = call "CRYGet Difference Array.vi"("Array 2"=w840, "Array 1"=w843) -> ("Diff Out"=w844:i32[])  [unwired: 3 in, 6 out]
                  n234 = call "CRYSymbol Conversion.vi"("nDatas"=w844, "sActin"="SUBTRACT") -> ()  [unwired: 10 in]
                }
                frame False {
                  n235 = Index Array(array=w874) -> (element=w873:i32)  [unwired: 1 in]
                  n236 = Search 1D Array(1D array=w870, element=w873) -> (index of element=w871:i32)  [unwired: 1 in]
                  n237 = Build Array(w871) -> (w868:i32[])
                  n238 = invoke class="VI" method="Ctrl Val.Set"(reference=w867, "Control Name"="SelectedRow", "Value"=w868) -> (reference out=w878:refnum<vi>)  [unwired: 2 in, 4 out]
                  n239 = Delete From Array(array=w870, index=w871) -> (array with subset deleted=w869:i32[])  [unwired: 1 in, 1 out]
                  n240 = call "CRYGet Two Units Rows.vi"("pGraph VI In"=w867, "Old Rows In"=w869) -> ("Two Units"=w881:i32)  [unwired: 3 in, 6 out]
                  n241 = call "CRYGet Boolean Reference.vi"("Label Name"="RemoveSome", "VI Refnum"=w878) -> ("Boolean Ref"=w876:refnum<vi>)  [unwired: 7 in, 2 out]
                  n242 = property class="Bool"(reference=w876, "Val(Sgnl)"=TRUE) -> ()  [unwired: 1 in, 2 out]
                }
              }
            }
            frame False {
              n243 = call "CRYGet Difference Array.vi"("Array 2"=w886, "Array 1"=w887) -> ("Diff Out"=w888:i32[])  [unwired: 3 in, 6 out]
              n244 = call "CRYGet Two Units Rows.vi"("pGraph VI In"=w882, "New Rows In"=w888, "Old Rows In"=w886) -> ("Two Units"=w885:i32, "New Rows Out"=w889:i32[], "New Exist?"=w890:bool)  [unwired: 2 in, 4 out]
              n245 = case shown="True" w890 {
                tunnel: w891 -> [_ w902]
                tunnel: w889 -> [_ w896]
                tunnel: ["NONE" ("sActin") w898] -> w884
                tunnel: [i32[] [] ("All Rows Out") w897] -> w883
                tunnel: w882 -> [_ w894]
                frame False {
                }
                frame True {
                  n246 = call "CRYPlot Octave Graph.vi"("pGraph VI In"=w894, "Selected Rows In"=w896) -> ("Color Info"=w901:u32[], "Curve Name"=w900:string[], "All Rows Out"=w899:i32[], "ItemSyms"=w895:i32[])  [unwired: 6 in]
                  n247 = call "CRYData View Legend New Insert.vi"("Item Symbols"=w895, "Color Array"=w901, "ItemName Array"=w900, "pGraph VI In"=w894) -> ()  [unwired: 1 in, 7 out]
                  n248 = case shown="False" w902 {
                    tunnel: w896 -> [w903 _]
                    tunnel: w899 -> [_ w906]
                    tunnel: ["APPEND" ("sActin") "ACTIVE" ("sActin")] -> w898
                    tunnel: [w903 w906] -> w897
                    frame True {
                    }
                    frame False {
                    }
                  }
                }
              }
            }
          }
        }
        frame Default {
        }
      }
      n249 = call "CRYSymbol Conversion.vi"("CurLib Tab Type"=w134, "nDatas"=w128, "sData"="TAB_CHANGE" ("sActin"), "sActin"=w129) -> ()  [unwired: 8 in]
      n250 = case shown="\"OCTAVE\", \"WAVE\", \"XY\"" w122 {
        tunnel: w118 -> [_ w140]
        tunnel: w130 -> [_ w139]
        frame Default {
        }
        frame "OCTAVE", "WAVE", "XY" {
          n251 = call "CRYGet Numeric Reference.vi"("Label Name"="Repaint Watermark" ("Control Name"), "VI Refnum"=w140) -> ("Numeric Ref Out"=w142:refnum<vi>)  [unwired: 9 out]
          n252 = property class="DigNum"(reference=w142, "Val(Sgnl)"=w139) -> ()  [unwired: 1 in, 2 out]
        }
      }
    }
  }
